vi "OCT with WavePond Clock periodic save.vi"() -> ()   [LabVIEW 2014]
doc: "I. Description:\nThis example demonstrates how to acquire a continuous amount of data (Waveform) using the DAQ device's internal clock.\n\nII. Instructions for Running:\n1. Create an analog input voltage channel.\n2. Set the rate for the sample clock. Additionally, define the sample mode to be continuous.\n3. Call the Start VI to start the acquisition.\n4. Read the waveform data in a loop until the user hits the stop button or an error occurs.\nNote: This example reads data from one or more channels and returns an array of data. Use the Index Array function to access an individual channel of data.\n5. Call the Clear Task VI to clear the Task.\n6. Use the popup dialog box to display an error if any.\n\nIV. I/O Connections Overview:\nMake sure your signal input terminal matches the Physical Channel I/O Control. For further connection information, refer to your hardware reference manual."
uses:
  ATS-VI/ATS_ctl/Device_Ctrl.ctl
  ATS-VI/ATS_ctl/ATS_Async_Ctrl.ctl
  ATS-VI/ATS_ctl/ATS_Async_Mode.ctl
  ATS-VI/ATS_ctl/ATS_DMA_Channel.ctl
  ATS-VI/ATS_ctl/ATS_ReadSamples.ctl
  ATS-VI/ATS_ctl/ATS_Check_Ctrl.ctl
  ATS-VI/ATS_ctl/ClockSource.ctl
  Galvo VIs/galvo_states.ctl
  Signal Processing/processing_states.ctl
  En Face/En Face States.ctl
  Saving Data/Saving Data States.ctl
  Type Defs/OCT Hardware States.ctl
  ATS-VI/ATS_ctl/Range.ctl
  ATS-VI/ATS_ctl/Impedance.ctl
  Type Defs/OCT Imaging Parameters Cluster.ctl
  Signal Processing/Display Raw Data states.ctl
  ATS-VI/ATS_ctl/ATS_Spec_Selector.ctl
  Classes/Galvo/Scanning Cluster.ctl
  Classes/Galvo/Galvo.lvclass
  Type Defs/OCT DAQ Channel Data Type.ctl
  Type Defs/Display States.ctl
  ATS-VI/ATS_ctl/Coupling.ctl
  ATS-VI/ATS_ctl/Bandwidth.ctl
  ATS-VI/ATS_ctl/InputCtrl.ctl
  ATS-VI/ATS_ctl/TriggerEngine.ctl
  ATS-VI/ATS_ctl/ExtTrigRange.ctl
  ATS-VI/ATS_ctl/ExtTrigger.ctl
  ATS-VI/ATS_ctl/TriggerOperation.ctl
  ATS-VI/ATS_ctl/Trigger.ctl
  ATS-VI/ATS_ctl/ClockRate.ctl
  ATS-VI/ATS_ctl/ClockEdge.ctl
  ATS-VI/ATS_ctl/Clock.ctl
  ATS-VI/ATS_ctl/Record.ctl
  ATS-VI/ATS_ctl/ATS_Global.ctl
  ATS-VI/ATS_ctl/ATS_Async_Status.ctl
  En Face/En Face Depth Parameters.ctl
  ATS-VI/ATS_ctl/ATS_Async_Setting.ctl
panel:
  in  "update en face image?":bool
  in  "total measurement time":dbl
  in  "save every ? second":dbl
  out "First Time?":bool
  out "Save Data":bool
  in  "Async_Setting":T1
  out "Processing Finished":bool
  in  "OCT Hardware States":T2=enum."Save Sweep"
  out "Save State":T3=enum."Initialize"
  out "Clock Length":u32=6304
  out "Reset DAQ":bool
  in  "Tab Control":T4(tab)
  in  "B-Scans Per Buffer":i32=4
  out "Async_Status":T5
  out "Current State":T2=enum."Set Resampling Array"
  in  "Channels":tag="Dev1/ao0:1"
  in  "Trigger Source":tag="/Dev1/PFI7"
  in  "Imaging Parameters":T6={"Points Per A-Scan"=0, "A-Scans per B-Scan"=0, "Voltage Range"=1.0, "Card Resolution (bits)"=12}
  in  "Setup_In":T7={"Record"={"Count"=1, "Presize"=0, "Length"=1408}, "Clock"={"ClckSource"=enum."External", "ClckRate"=17, "ClckEdge"=0, "Decimation"=0}, "Input A"={"Coupling"=enum."DC", "Range"=3, "Impedance"=enum."50 ohms", "Bandwidth"=enum."Full Bandwidth"}, "Input B"={"Coupling"=enum."DC", "Range"=3, "Impedance"=enum."50 ohms", "Bandwidth"=enum."Full Bandwidth"}, "Trigger"={"TrigOperation"=enum."Only X", "Timeout (s)"=1.0, "Trig. Delay"=0, "Engine X"={"Source"=enum."External", "Slope"=enum."Positive", "Level"=150}, "Engine Y"={"Source"=enum."Disable", "Slope"=enum."Positive", "Level"=128}, "ExtTrigControl"={"Coupling"=enum."DC", "Range"=enum."TTL"}}} {"Clock"."ClckEdge" items=["Rising", "Falling"]; "Clock"."ClckRate" items=["1 kS/s", "2 kS/s", "5 kS/s", "10 kS/s", "20 kS/s", "50 kS/s", "100 kS/s", "200 kS/s", "500 kS/s", "1 MS/s", "2 MS/s", "5 MS/s", "10 MS/s", "20 MS/s", "50 MS/s", "100 MS/s", "125 MS/s", "160 MS/s", "180 MS/s"]; "Input B"."Range" items=["200mV", "400mV", "800mV", "2 V", "4 V", "8 V", "16 V"]; "Trigger"."Timeout (s)" format="%.2f"; "Input A"."Range" items=["200mV", "400mV", "800mV", "2 V", "4 V", "8 V", "16 V"]}
  in  "OK Button":bool
  in  "Data Format":T23
  out "Channel A or B Phase (or Channel B Raw)":sgl[][](graph)
  out "Channel A or B Intensity (or Channel A Raw)":sgl[][](graph)
  in  "Display":T24
  out "En Face":dbl[][](graph)
  in  "En Face Parameters":T25={"En Face Start\nDepth"=50, "En Face End\nDepth"=200}
  in  "Save Sweep":bool
  in  "Scanning":T26={"Fast Axis Offset"=300.0, "Slow Axis Offset"=1.0, "Slow Axis Amp"=8.0, "Fast Axis Amp"=8.0, "B-scans (rings)"=1, "A(cluster)/B"=0, "Scan Pattern"=enum."Raster"} {"A(cluster)/B" max=1000 step=1; "B-scans (rings)" max=1000 step=1; "Fast Axis Amp" max=20 format="%#.2f"; "Slow Axis Amp" max=20 format="%#.2f"; "Slow Axis Offset" max=10 format="%#.2f"; "Fast Axis Offset" max=10 format="%#.2f"}
  in  "Stop Button":bool
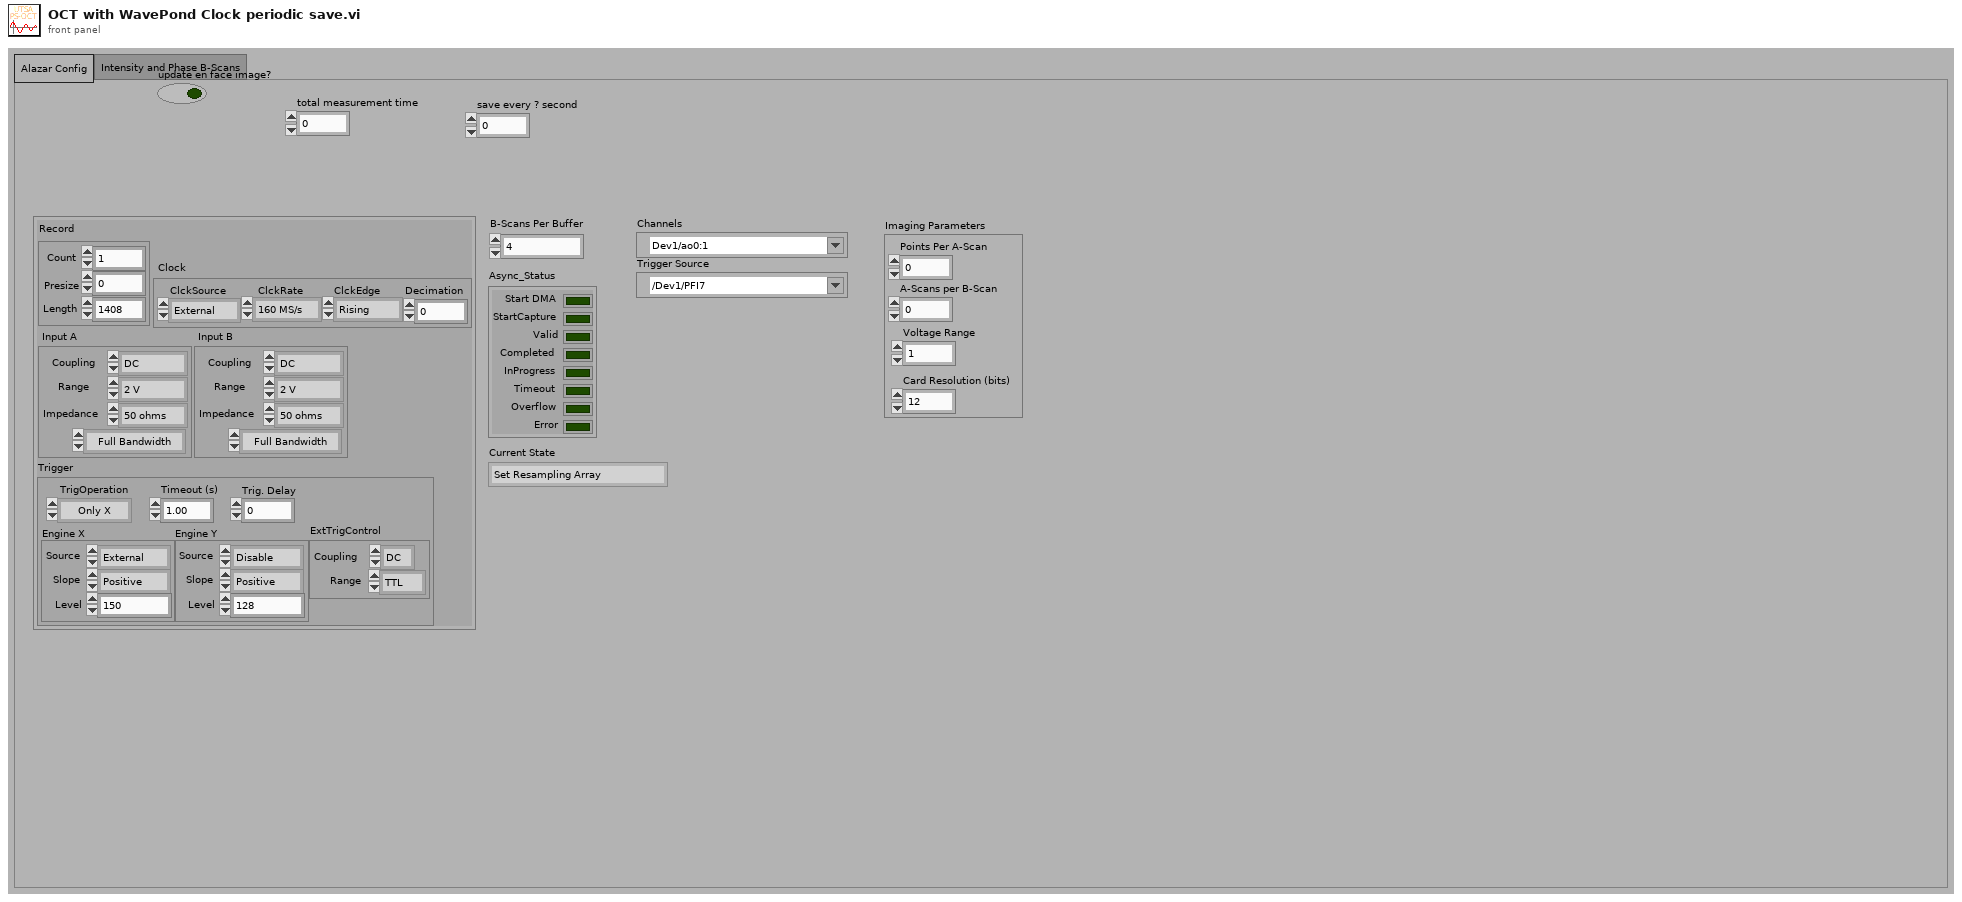
[diagram p1: front panel]
types:
  T1 = typedef "ATS_Async_Setting.ctl" = cluster{"UseHeader":u32, "Rec/Buffer":u32, "Total_Rec":u32, "DataBuffer":bool, "GetProcessedData":bool}
  T2 = typedef "OCT Hardware States.ctl" = enum16{"Acquire Data", "Initialize Laser", "Initialize Galvos", "Startup", "Reset DAQ", "Background Subtraction", "Acquire Background", "Update DAQ Parameters", "Stop", "Set Clock", "Initialize DAQ", "Set Resampling Array", "Save Sweep", "Configure Laser", "128 x 128", "512 x 512", "Review Data"}
  T3 = typedef "Saving Data States.ctl" = enum16{"Get Queue Size", "Get Queue", "Get Timeout", "Flush Queue", "Close Files", "Create Files", "Do Nothing", "Initialize", "Enqueue Data", "Save Data", "Shutdown"}
  T4 = enum32{"Alazar Config", "Intensity and Phase B-Scans"}
  T5 = typedef "ATS_Async_Status.ctl" = cluster{"Start DMA":bool, "StartCapture":bool, "Valid":bool, "Completed":bool, "InProgress":bool, "Timeout":bool, "Overflow":bool, "Error":bool}
  T6 = typedef "OCT Imaging Parameters Cluster.ctl" = cluster{"Points Per A-Scan":i32, "A-Scans per B-Scan":i32, "Voltage Range":sgl, "Card Resolution (bits)":u16}
  T7 = typedef "ATS_Global.ctl" = cluster{"Record":T8, "Clock":T9, "Input A":T13, "Input B":T13, "Trigger":T18}
  T8 = typedef "Record.ctl" = cluster{"Count":u32, "Presize":u32, "Length":u32}
  T9 = typedef "Clock.ctl" = cluster{"ClckSource":T10, "ClckRate":T11, "ClckEdge":T12, "Decimation":u32}
  T10 = typedef "ClockSource.ctl" = enum16{"Internal", "External", "Medium Ext.", "Slow Ext.", "Ext. AC", "Ext. DC", "Ext. (PLL)"}
  T11 = typedef "ClockRate.ctl" = u32
  T12 = typedef "ClockEdge.ctl" = u16
  T13 = typedef "InputCtrl.ctl" = cluster{"Coupling":T14, "Range":T15, "Impedance":T16, "Bandwidth":T17}
  T14 = typedef "Coupling.ctl" = enum16{"AC", "DC"}
  T15 = typedef "Range.ctl" = u32
  T16 = typedef "Impedance.ctl" = enum16{"1M ohms", "50 ohms"}
  T17 = typedef "Bandwidth.ctl" = enum16{"Full Bandwidth", "Reduce Bandwidth"}
  T18 = typedef "Trigger.ctl" = cluster{"TrigOperation":T19, "Timeout (s)":dbl, "Trig. Delay":u32, "Engine X":T20, "Engine Y":T20, "ExtTrigControl":T21}
  T19 = typedef "TriggerOperation.ctl" = enum16{"Only X", "Only Y", "X or Y", "X and Y", "X xor Y", "X and not Y", "not X and Y"}
  T20 = typedef "TriggerEngine.ctl" = cluster{"Source":enum32{"Chan_A", "Chan_B", "External", "Disable"}, "Slope":enum32{"Positive", "Negative"}, "Level":u32}
  T21 = typedef "ExtTrigger.ctl" = cluster{"Coupling":T14, "Range":T22}
  T22 = typedef "ExtTrigRange.ctl" = enum16{"1 V", "5 V", "TTL"}
  T23 = typedef "OCT DAQ Channel Data Type.ctl" = enum16{"Channel 1", "Channel 2", "Channel 1 and 2"}
  T24 = typedef "Display States.ctl" = enum16{"Channel A", "Channel B"}
  T25 = typedef "En Face Depth Parameters.ctl" = cluster{"En Face Start\nDepth":i32, "En Face End\nDepth":i32}
  T26 = typedef "Galvo.lvclass/Scanning Cluster.ctl" = cluster{"Fast Axis Offset":sgl, "Slow Axis Offset":sgl, "Slow Axis Amp":sgl, "Fast Axis Amp":sgl, "B-scans (rings)":u32, "A(cluster)/B":u32, "Scan Pattern":enum16{"Raster"}}
  T27 = typedef "ATS_Check_Ctrl.ctl" = enum16{"None", "NO_ATS9462", "ATS9462_Traditional", "Verify Board", "OnBoard Memory", "Board & Memory", "Master/Slave", "NO Master/Slave"}
  T28 = typedef "Device_Ctrl.ctl" = enum16{"Status", "About", "Arm", "ForceTrig", "Abort", "Initialize", "Init (NoPreset)", "Info", "Close", "Calibrate", "SetManually", "LED_ON", "LED_OFF"}
  T29 = typedef "ATS_Spec_Selector.ctl" = enum16{"None", "ClckSource", "ClckEdge", "ClckRate", "InputRange", "InputCoupling", "Impedance", "Bandwidth", "AsyncDMA", "Memory", "ExtTrigCoupling", "ExtTrigRange", "AUX_IO_Trig", "AUX_IO_Slope", "Trigger_Source"}
  T30 = typedef "galvo_states.ctl" = enum16{"Reset", "Reset Galvos?", "Center Galvos", "Register Callback", "Get Scan Parameters", "Show", "Initialize", "Run Raster", "Load Raster", "Run Circle", "Shutdown"}
  T31 = typedef "processing_states.ctl" = enum16{"Initialize", "Set Background", "Update Imaging Parameters", "Get Queue", "Process Data", "Get Size", "Flush Data", "Set Reample Array", "Get Last Processed BScan", "Shutdown"}
  T32 = typedef "Display Raw Data states.ctl" = enum16{"Add Raw", "Add Processed", "Show"}
  T33 = typedef "En Face States.ctl" = enum16{"Save BMP", "Show", "Clear En Face", "Update EnFace"}
  T34 = typedef "Processed OCT Data.ctl" = cluster{"Intensity A":sgl[][][], "Phase A":sgl[][][], "Intensity B":sgl[][][], "Phase B":sgl[][][]}
  T35 = enum8{"Enabled", "Disabled", "Disabled and Grayed Out"}
  T36 = typedef "ATS_Async_Ctrl.ctl" = enum16{"SetupDMA", "StartCapture", "Get", "Get_Stream", "Abort", "Stop"}
  T37 = typedef "ATS_ReadSamples.ctl" = cluster{"Offset":i32, "Length":u32}
  T38 = typedef "ATS_DMA_Channel.ctl" = enum16{"Channel_A", "Channel_B", "A & B"}
  T39 = typedef "ATS_Async_Mode.ctl" = enum16{"Continuous", "Triggered", "No-Pre-Trigger", "Traditional"}
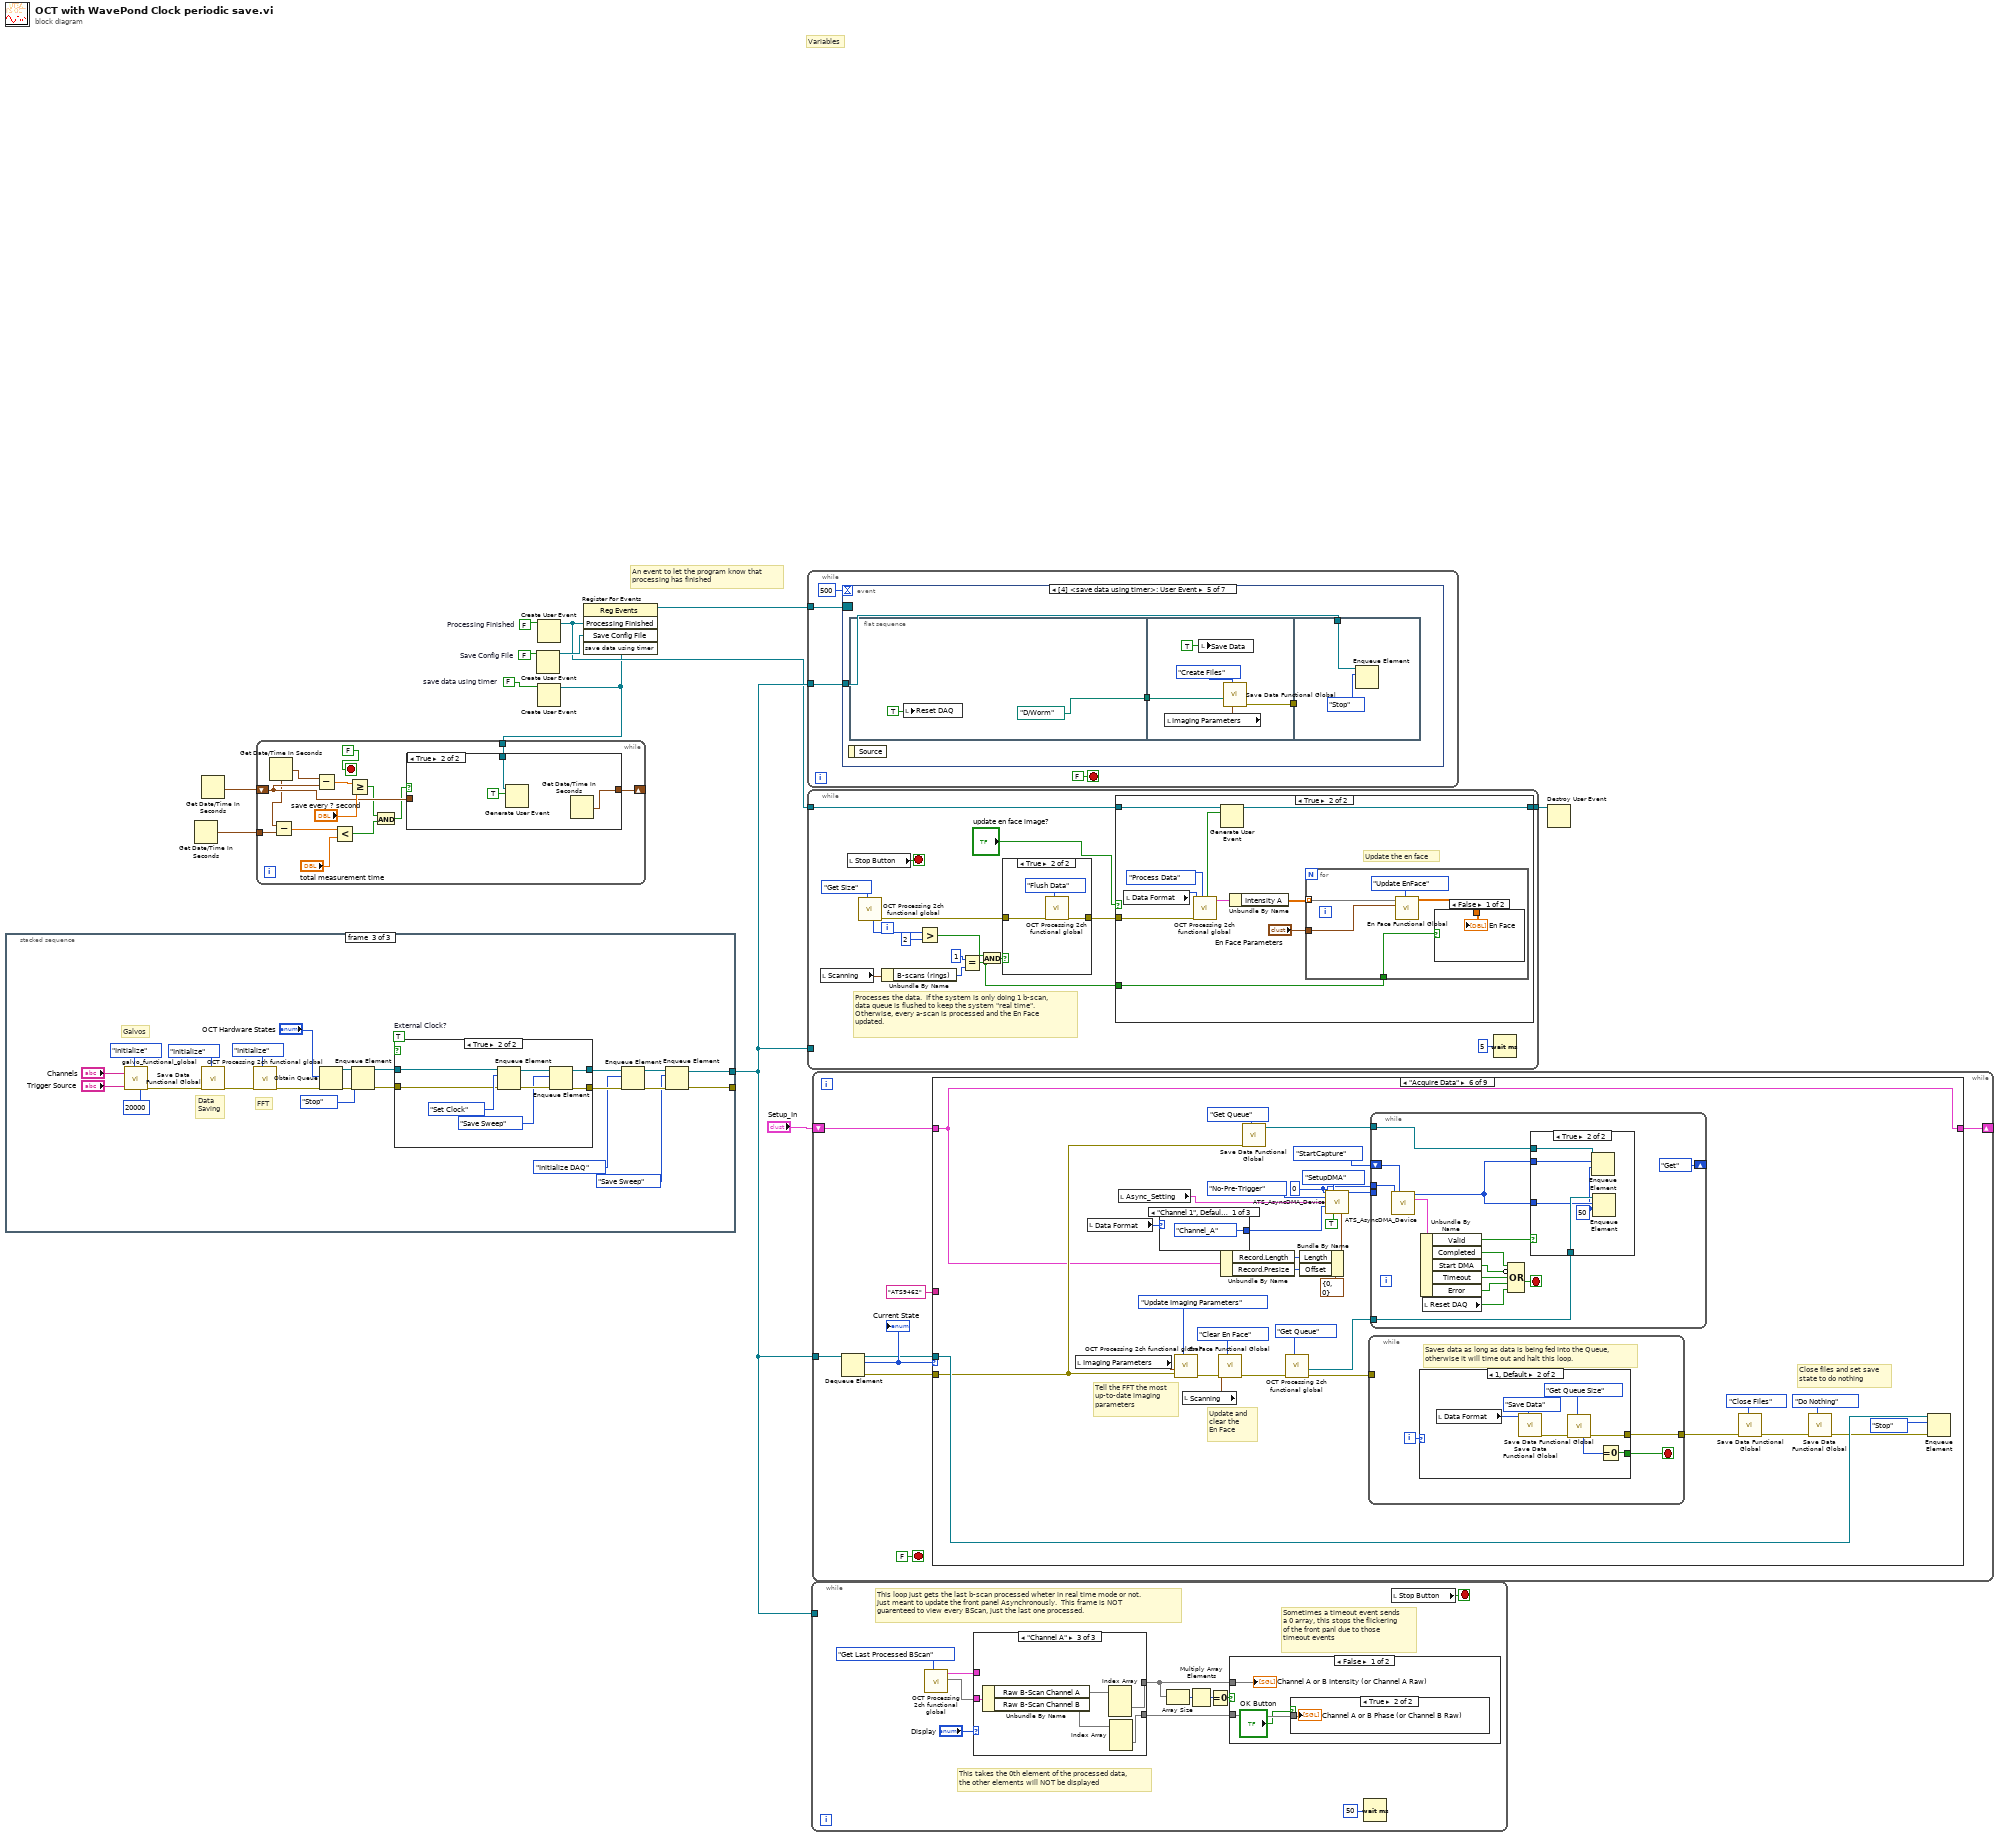
[diagram p0: block diagram]
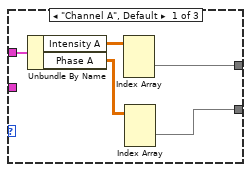
[diagram p8: hidden frame]
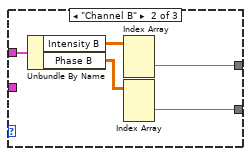
[diagram p9: hidden frame]
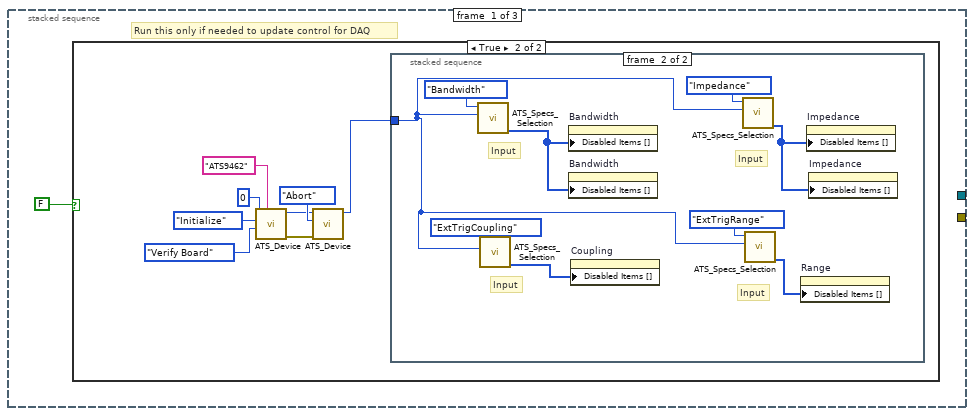
[diagram p10: hidden frame]
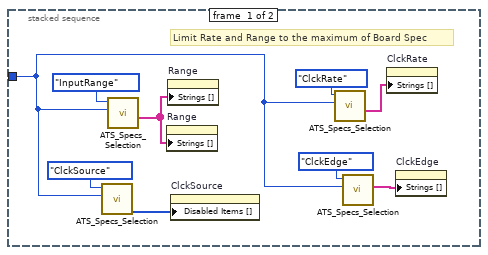
[diagram p12: hidden frame]
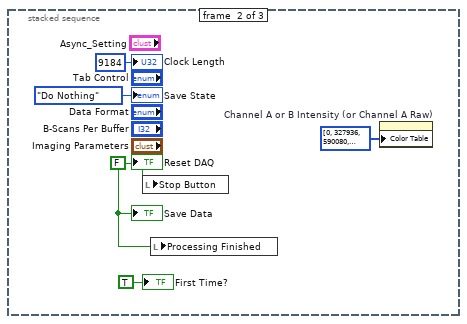
[diagram p13: hidden frame]
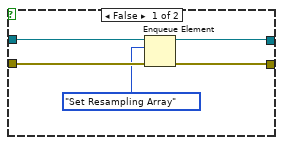
[diagram p14: hidden frame]
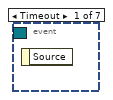
[diagram p15: hidden frame]
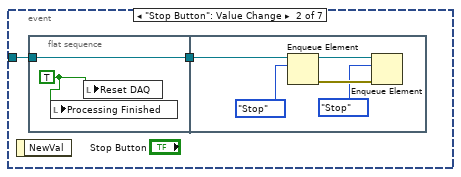
[diagram p16: hidden frame]
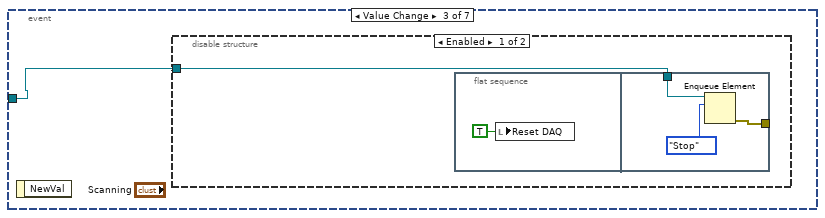
[diagram p17: hidden frame]
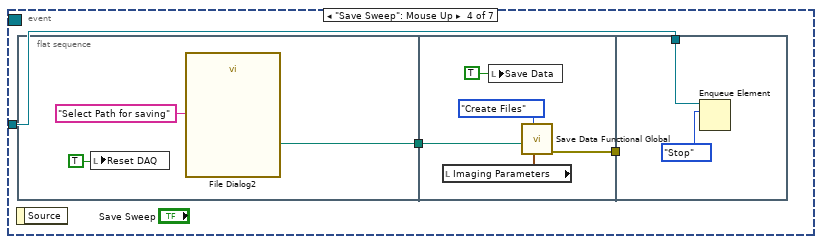
[diagram p19: hidden frame]
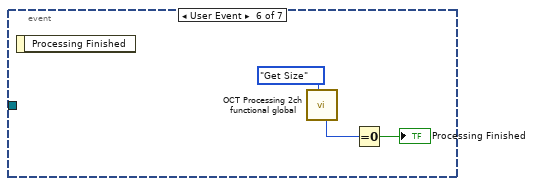
[diagram p20: hidden frame]
diagram:
  w3 = FALSE  # save data using timer
  w4 = FALSE  # Save Config File
  w12 = FALSE  # Processing Finished
  # "An event to let the program know that\nprocessing has finished"
  # "Variables"
  n1 = stacked-sequence {
    tunnel: [_ _ w58] -> _
    tunnel: [_ _ w64] -> w9
    frame #0 {
      # "Run this only if needed to update control for DAQ"
      n2 = case shown="True" FALSE {
        frame False {
        }
        frame True {
          n3 = call "ATS_Device.vi"("BoardToVerify"="ATS9462", "ATS_Check"=ATS_Check_Ctrl."Verify Board", "DevCtrl"=Device_Ctrl."Initialize", "DeviceIn"=0 ("Device")) -> ("error out"=w17:errorcluster, "DeviceOut"=w19:i32)  [unwired: 1 in, 5 out]
          n4 = call "ATS_Device.vi"("error in (no error)"=w17, "DevCtrl"=Device_Ctrl."Abort", "DeviceIn"=w19) -> ("DeviceOut"=w15:i32)  [unwired: 2 in, 6 out]
          n5 = stacked-sequence {
            tunnel: w15 -> [w24 w31]
            frame #0 {
              # "Limit Rate and Range to the maximum of Board Spec"
              n6 = call "ATS_Specs_Selection.vi"("Device"=w24, "ATS_Spec_Selector"=ATS_Spec_Selector."ClckSource") -> ("Disabled_Item"=w23:i32[])  [unwired: 3 in, 6 out]
              n7 = call "ATS_Specs_Selection.vi"("Device"=w24, "ATS_Spec_Selector"=ATS_Spec_Selector."InputRange") -> ("Possible_Item"=w30:string[])  [unwired: 3 in, 6 out]
              n8 = property on="Range" class="Ring (strict)"("Strings []"=w30) -> ()  [unwired: 2 in, 2 out]
              n9 = property on="Range" class="Ring (strict)"("Strings []"=w30) -> ()  [unwired: 2 in, 2 out]
              n10 = property on="ClckSource" class="Enum (strict)"("Disabled Items []"=w23) -> ()  [unwired: 2 in, 2 out]
              n11 = call "ATS_Specs_Selection.vi"("Device"=w24, "ATS_Spec_Selector"=ATS_Spec_Selector."ClckRate") -> ("Possible_Item"=w28:string[])  [unwired: 3 in, 6 out]
              n12 = call "ATS_Specs_Selection.vi"("Device"=w24, "ATS_Spec_Selector"=ATS_Spec_Selector."ClckEdge") -> ("All_Item"=w22:string[])  [unwired: 3 in, 6 out]
              n13 = property on="ClckRate" class="Ring (strict)"("Strings []"=w28) -> ()  [unwired: 2 in, 2 out]
              n14 = property on="ClckEdge" class="Ring (strict)"("Strings []"=w22) -> ()  [unwired: 2 in, 2 out]
            }
            frame #1 {
              # "Input"
              # "Input"
              # "Input"
              # "Input"
              n15 = call "ATS_Specs_Selection.vi"("Device"=w31, "ATS_Spec_Selector"=ATS_Spec_Selector."Bandwidth") -> ("Disabled_Item"=w37:i32[])  [unwired: 3 in, 6 out]
              n16 = call "ATS_Specs_Selection.vi"("Device"=w31, "ATS_Spec_Selector"=ATS_Spec_Selector."ExtTrigCoupling") -> ("Disabled_Item"=w33:i32[])  [unwired: 3 in, 6 out]
              n17 = property on="Bandwidth" class="Enum (strict)"("Disabled Items []"=w37) -> ()  [unwired: 2 in, 2 out]
              n18 = property on="Bandwidth" class="Enum (strict)"("Disabled Items []"=w37) -> ()  [unwired: 2 in, 2 out]
              n19 = property on="Coupling" class="Enum (strict)"("Disabled Items []"=w33) -> ()  [unwired: 2 in, 2 out]
              n20 = call "ATS_Specs_Selection.vi"("Device"=w31, "ATS_Spec_Selector"=ATS_Spec_Selector."Impedance") -> ("Disabled_Item"=w36:i32[])  [unwired: 3 in, 6 out]
              n21 = call "ATS_Specs_Selection.vi"("Device"=w31, "ATS_Spec_Selector"=ATS_Spec_Selector."ExtTrigRange") -> ("Disabled_Item"=w32:i32[])  [unwired: 3 in, 6 out]
              n22 = property on="Range" class="Enum (strict)"("Disabled Items []"=w32) -> ()  [unwired: 2 in, 2 out]
              n23 = property on="Impedance" class="Enum (strict)"("Disabled Items []"=w36) -> ()  [unwired: 2 in, 2 out]
              n24 = property on="Impedance" class="Enum (strict)"("Disabled Items []"=w36) -> ()  [unwired: 2 in, 2 out]
            }
          }
        }
      }
    }
    frame #1 {
      w41 = FALSE ("Sweep Ready for saving")
      n25 = local write "Stop Button"(w41) -> ()
      n26 = local write "Processing Finished"(w41) -> ()
      n27 = property on="Channel A or B Intensity (or Channel A Raw)" class="IntGraph (strict)"("Color Table"=u32[] [0, 327936, 590080, 852224, 983296, 1114624, 1180160, 1311232, 1442304, 1573632, 1704704, 1770240, 1901312, 1966848, 2098176, 2163712, 2294784, 2491392, 2557184, 2688256, 2753792, 2884864, 2950656, 3081728, 3147264, 3344129, 3475457, 3540993, 3672321, 3738113, 3869185, 3934977, 4066305, 4197633, 4328961, 4394497, 4460289, 4591617, 4657409, 4788481, 4854273, 4985601, 5116929, 5248257, 5314049, 5379841, 5511169, 5576961, 5708033, 5773825, 5905153, 6036482, 6167810, 6233346, 6299138, 6430466, 6496258, 6562050, 6693634, 6759426, 6890754, 7022082, 7087874, 7153666, 7284994, 7350786, 7482114, 7547906, 7613698, 7745026, 7876354, 8007682, 8073474, 8139522, 8205314, 8336642, 8467970, 8533763, 8599555, 8665347, 8731139, 8862467, 8993795, 9059587, 9125380, 9191428, 9257220, 9388548, 9454340, 9520132, 9585924, 9717253, 9848837, 9914629, 9980165, 10045957, 10177541, 10243334, 10309126, 10375174, 10440966, 10572294, 10703623, 10769416, 10835208, 10901256, 10967049, 11033097, 11033609, 11099401, 11165450, 11231242, 11231754, 11297547, 11363339, 11429131, 11495180, 11495692, 11561740, 11693069, 11758861, 11759373, 11825165, 11891214, 11957006, 12022799, 12023311, 12089103, 12220944, 12286736, 12286736, 12352529, 12418577, 12484370, 12550162, 12615954, 12681747, 12747796, 12813588, 12813845, 12879894, 12945686, 13077015, 13142808, 13143064, 13208856, 13274905, 13340697, 13340953, 13472282, 13538075, 13604379, 13670172, 13735964, 13801757, 13867550, 13933343, 13999392, 13999648, 14065441, 14131234, 14197027, 14197541, 14263334, 14329383, 14395176, 14460969, 14592553, 14658346, 14724139, 14789932, 14790189, 14856238, 14922287, 14988080, 15053873, 15054130, 15119923, 15185972, 15251765, 15317559, 15383353, 15449146, 15449660, 15515454, 15515968, 15516226, 15582021, 15582278, 15582536, 15648587, 15648844, 15714639, 15714897, 15715155, 15780949, 15781463, 15847256, 15847770, 15848028, 15913823, 15914081, 15979875, 15980133, 15980391, 16046441, 16046444, 16046703, 16046705, 16112500, 16113015, 16113274, 16113277, 16179072, 16179330, 16179588, 16245384, 16245387, 16245389, 16245648, 16311443, 16376982, 16377241, 16377499, 16443294, 16443553, 16443555, 16443815, 16509866, 16510124, 16510127, 16575923, 16575924, 16576182, 16576441, 16576443, 16576702, 16576705, 16576963, 16577222, 16577224, 16577482, 16577485, 16577743, 16577745, 16578004, 16578262, 16578264, 16578523, 16578782, 16579040, 16579299, 16579301, 16579303, 16579562, 16579821]) -> ()  [unwired: 2 in, 2 out]
      "Clock Length" <- u32 9184 ("Clock Length")
      "Save State" <- Saving_Data_States."Do Nothing" ("Save State")
      "Reset DAQ" <- w41
      "Save Data" <- w41
      "First Time?" <- TRUE ("First Time?")
    }
    frame #2 {
      w46 = TRUE  # External Clock?
      # "FFT"
      # "Data \nSaving"
      # "Galvos"
      n28 = call "galvo_functional_global.vi"(4:20000 ("Sweep Speed"), "State"=galvo_states."Initialize", "Trigger Source"="Trigger Source", "Analog Output"="Channels") -> ("error out"=w55:errorcluster)  [unwired: 6 in, 1 out]
      n29 = call "Save Data Functional Global.vi"("States"=Saving_Data_States."Initialize", "error in (no error)"=w55) -> ("error out"=w60:errorcluster)  [unwired: 6 in, 3 out]
      n30 = call "OCT Processing 2ch functional global.vi"("State"=processing_states."Initialize", "error in (no error)"=w60) -> ("error out"=w61:errorcluster)  [unwired: 5 in, 4 out]
      n31 = Obtain Queue(element data type="OCT Hardware States", error in (no error)=w61) -> (queue out=w49:refnum<queue>, error out=w48:errorcluster)  [unwired: 3 in, 1 out]
      n32 = Enqueue Element(queue=w49, element=OCT_Hardware_States."Stop", error in (no error)=w48) -> (queue out=w51:refnum<queue>, error out=w50:errorcluster)  [unwired: 1 in, 1 out]
      n33 = case shown="True" w46 {
        tunnel: [w70 w79] -> w68
        tunnel: [w71 w78] -> w67
        tunnel: w51 -> [w73 w75]
        tunnel: w50 -> [w72 w74]
        frame False {
          n34 = Enqueue Element(queue=w73, element=OCT_Hardware_States."Set Resampling Array", error in (no error)=w72) -> (queue out=w70:refnum<queue>, error out=w71:errorcluster)  [unwired: 1 in, 1 out]
        }
        frame True {
          n35 = Enqueue Element(queue=w75, element=OCT_Hardware_States."Set Clock", error in (no error)=w74) -> (queue out=w81:refnum<queue>, error out=w80:errorcluster)  [unwired: 1 in, 1 out]
          n36 = Enqueue Element(queue=w81, element=OCT_Hardware_States."Save Sweep", error in (no error)=w80) -> (queue out=w79:refnum<queue>, error out=w78:errorcluster)  [unwired: 1 in, 1 out]
        }
      }
      n37 = Enqueue Element(queue=w68, element=OCT_Hardware_States."Initialize DAQ", error in (no error)=w67) -> (queue out=w66:refnum<queue>, error out=w65:errorcluster)  [unwired: 1 in, 1 out]
      n38 = Enqueue Element(queue=w66, element=OCT_Hardware_States."Save Sweep", error in (no error)=w65) -> (queue out=w64:refnum<queue>, error out=w58:errorcluster)  [unwired: 1 in, 1 out]
    }
  }
  n39 = Get Date/Time In Seconds() -> (seconds since 1Jan1904=w1:timestamp)
  n40 = Get Date/Time In Seconds() -> (seconds since 1Jan1904=w5:timestamp)
  n41 = Create User Event(user event datatype=w4) -> (user event=w8:refnum<user-event>)  [unwired: 1 in, 1 out]
  n42 = Create User Event(user event datatype=w12) -> (user event=w7:refnum<user-event>)  [unwired: 1 in, 1 out]
  n43 = Create User Event(user event datatype=w3) -> (user event=w2:refnum<user-event>)  [unwired: 1 in, 1 out]
  n44 = while {
    shift-right: [w91] -> _
    shift-left: w5 -> [w90]
    tunnel: w2 -> [w89]
    tunnel: w1 -> [w87]
    stop <- FALSE stop-if-true
    n45 = Get Date/Time In Seconds() -> (seconds since 1Jan1904=w86:timestamp)
    n46 = Subtract(x=w86, y=w87) -> (x-y=w85:dbl)
    n47 = Subtract(x=w86, y=w90) -> (x-y=w93:dbl)
    n48 = Less?(x=w85, y="total measurement time") -> (x < y?=w84:bool)
    n49 = Greater Or Equal?(x=w93, y="save every ? second") -> (x >= y?=w83:bool)
    n50 = And(x=w83, y=w84) -> (x .and. y?=w82:bool)
    n51 = case shown="True" w82 {
      tunnel: [w95 w98] -> w91
      tunnel: w90 -> [w95 _]
      tunnel: w89 -> [_ w97]
      frame False {
      }
      frame True {
        n52 = Generate User Event(user event=w97, event data cluster=TRUE ("event data")) -> ()  [unwired: 2 in, 2 out]
        n53 = Get Date/Time In Seconds() -> (seconds since 1Jan1904=w98:timestamp)
      }
    }
  }
  n54 = register-events(w7, w8, w2) -> (reference out=w11:refnum<event-registration>)  [unwired: 2 in, 1 out]
  n55 = while {
    tunnel: w9 -> [w100]
    tunnel: w11 -> [w101]
    stop <- FALSE stop-if-true
    n56 = event shown="[4] <save data using timer>: User Event" {
      selector: w101 -> [_ _ _ _ _ _ _]
      dyn-events: _ -> [_ _ _ _ _ _ _]
      timeout: 500 -> [_ _ _ _ _ _ _]
      tunnel: w100 -> [_ w103 w112 w120 w133 _ _]
      event Timeout {
        n57 = event-data() -> ()  [unwired: 1 in, 1 out]
      }
      event "Stop Button": Value Change {
        n58 = event-data() -> ()  [unwired: 1 in, 1 out]
        n59 = flat-sequence {
          tunnel: w103 -> [w106]
          tunnel: [w106] -> w104
          tunnel: w104 -> [w111]
          frame #0 {
            w105 = TRUE ("Reset DAQ")
            n60 = local write "Processing Finished"(w105) -> ()
            n61 = local write "Reset DAQ"(w105) -> ()
          }
          frame #1 {
            n62 = Enqueue Element(queue=w111, element=OCT_Hardware_States."Stop") -> (queue out=w108:refnum<queue>, error out=w109:errorcluster)  [unwired: 2 in, 1 out]
            n63 = Enqueue Element(queue=w108, element=OCT_Hardware_States."Stop", error in (no error)=w109) -> ()  [unwired: 1 in, 3 out]
          }
        }
      }
      event Value Change {
        n64 = event-data() -> ()  [unwired: 1 in, 1 out]
        n65 = disable-structure shown="Enabled" {
          disable-tunnel: w112 -> [w113 _]
          frame Enabled {
            n66 = flat-sequence {
              tunnel: w113 -> [w116]
              tunnel: [w115] -> _
              frame #0 {
                n67 = local write "Reset DAQ"(TRUE ("Reset DAQ")) -> ()
              }
              frame #1 {
                n68 = Enqueue Element(queue=w116, element=OCT_Hardware_States."Stop") -> (error out=w115:errorcluster)  [unwired: 2 in, 2 out]
              }
            }
          }
          frame Disabled {
          }
        }
      }
      event "Save Sweep": Mouse Up {
        n69 = event-data() -> ()  [unwired: 1 in, 1 out]
        n70 = flat-sequence {
          tunnel: [w121] -> w119
          tunnel: w119 -> [w128]
          tunnel: [w126] -> w118
          tunnel: w120 -> [w130]
          tunnel: w118 -> [_]
          frame #0 {
            n71 = local write "Reset DAQ"(TRUE ("Reset DAQ")) -> ()
            n72 = call "File Dialog2"("prompt"="Select Path for saving") -> ("selected path"=w121:path)  [unwired: 11 in, 3 out]
          }
          frame #1 {
            n73 = local read "Imaging Parameters"() -> (w125:T6)
            n74 = local write "Save Data"(TRUE ("Save Data")) -> ()
            n75 = call "Save Data Functional Global.vi"("Input Parameters"=w125, "States"=Saving_Data_States."Create Files", "Folder"=w128) -> ("error out"=w126:errorcluster)  [unwired: 5 in, 3 out]
          }
          frame #2 {
            n76 = Enqueue Element(queue=w130, element=OCT_Hardware_States."Stop") -> ()  [unwired: 2 in, 3 out]
          }
        }
      }
      event User Event {
        n77 = event-data() -> ()  [unwired: 1 in, 1 out]
        n78 = flat-sequence {
          tunnel: [path "D:/Worm" ("selected path")] -> w132
          tunnel: w132 -> [w140]
          tunnel: [w138] -> w131
          tunnel: w133 -> [w142]
          tunnel: w131 -> [_]
          frame #0 {
            n79 = local write "Reset DAQ"(TRUE ("Reset DAQ")) -> ()
          }
          frame #1 {
            n80 = local read "Imaging Parameters"() -> (w137:T6)
            n81 = local write "Save Data"(TRUE ("Save Data")) -> ()
            n82 = call "Save Data Functional Global.vi"("Input Parameters"=w137, "States"=Saving_Data_States."Create Files", "Folder"=w140) -> ("error out"=w138:errorcluster)  [unwired: 5 in, 3 out]
          }
          frame #2 {
            n83 = Enqueue Element(queue=w142, element=OCT_Hardware_States."Stop") -> ()  [unwired: 2 in, 3 out]
          }
        }
      }
      event User Event {
        n84 = event-data() -> ()  [unwired: 1 in, 1 out]
        n85 = call "OCT Processing 2ch functional global.vi"("State"=processing_states."Get Size") -> ("# elements in queue"=w144:i32)  [unwired: 6 in, 4 out]
        n86 = Equal To 0?(x=w144) -> (x = 0?=→"Processing Finished":bool)
      }
      event Menu Selection (User) {
        n87 = event-data() -> ("ItemTag"=w146:string)  [unwired: 1 in, 2 out]
        n88 = case shown="\"Raw Data\", Default" w146 {
          frame "Raw Data", Default {
            n89 = call "Display Raw Data.vi"("Enum"=Display_Raw_Data_states."Show") -> ()  [unwired: 11 in]
          }
        }
      }
    }
  }
  n90 = while {
    tunnel: w7 -> [w154]
    tunnel: [w153] -> w10
    tunnel: w9 -> [_]
    stop <- w163 stop-if-true
    # "Processes the data.  If the system is only doing 1 b-scan, \ndata queue is flushed to keep the system \"real time\".\nOtherwise, every a-scan is processed and the En Face\nupdated."
    n91 = local read "Scanning"() -> (w156:T26)
    n92 = local read "Stop Button"() -> (w163:bool)
    n93 = call "OCT Processing 2ch functional global.vi"("State"=processing_states."Get Size") -> ("error out"=w152:errorcluster, "# elements in queue"=w160:i32)  [unwired: 6 in, 3 out]
    n94 = Unbundle By Name(w156) -> ("B-scans (rings)"=w155:u32)
    n95 = Greater?(x=w160, y=2) -> (0:w161:bool)
    n96 = Equal?(x=u32 1, y=w155) -> (x = y?=w149:bool)
    n97 = And(x=w161, y=w149) -> (x .and. y?=w150:bool)
    n98 = case shown="True" w150 {
      tunnel: w152 -> [w181 w184]
      tunnel: [w181 w183] -> w151
      frame False {
      }
      frame True {
        n99 = call "OCT Processing 2ch functional global.vi"("State"=processing_states."Flush Data", "error in (no error)"=w184) -> ("error out"=w183:errorcluster)  [unwired: 5 in, 4 out]
      }
    }
    n100 = case shown="True" "update en face image?" {
      tunnel: w154 -> [w164 w171]
      tunnel: [w164 w169] -> w153
      tunnel: w151 -> [_ w166]
      tunnel: w149 -> [_ w165]
      frame False {
      }
      frame True {
        # "Update the en face"
        n101 = local read "Data Format"() -> (w172:T23)
        n102 = call "OCT Processing 2ch functional global.vi"("State"=processing_states."Process Data", "error in (no error)"=w166, "Data Format"=w172) -> ("Processed OCT Data"=w173:T34, "Time Out"=w170:bool)  [unwired: 4 in, 3 out]
        n103 = Generate User Event(user event=w171, event data cluster=w170) -> (user event out=w169:refnum<user-event>)  [unwired: 2 in, 1 out]
        n104 = Unbundle By Name(w173) -> ("Intensity A"=w167:sgl[][][])
        n105 = for {
          tunnel: "En Face Parameters" -> [w178]
          tunnel: w167 -> [w177] mode=indexing
          tunnel: w165 -> [w175]
          n106 = call "En Face Functional Global.vi"(7:En_Face_States."Update EnFace" ("En Face States"), 10:w178, "Intensity Graph 2"=w177) -> ("Intensity Graph"=w176:dbl[][])  [unwired: 7 in, 1 out]
          n107 = case shown="False" w175 {
            tunnel: w176 -> [w180 _]
            frame False {
              "En Face" <- w180
            }
            frame True {
            }
          }
        }
      }
    }
    n108 = Wait (ms)(milliseconds to wait=u32 5) -> ()  [unwired: 1 out]
  }
  n109 = while {
    tunnel: w9 -> [_]
    stop <- w195 stop-if-true
    # "Sometimes a timeout event sends\na 0 array, this stops the flickering\nof the front panl due to those \ntimeout events"
    # "This takes the 0th element of the processed data,\nthe other elements will NOT be displayed"
    # "This loop just gets the last b-scan processed wheter in real time mode or not. \nJust meant to update the front panel Asynchronously.  This frame is NOT\nguarenteed to view every BScan, just the last one processed."
    n110 = call "OCT Processing 2ch functional global.vi"("State"=processing_states."Get Last Processed BScan") -> (2:w191, "Processed OCT Data"=w189:T34)  [unwired: 5 in, 4 out]
    n111 = case shown="\"Raw Data A and B\"" "Display" {
      tunnel: w189 -> [w204 w205 _]
      tunnel: w191 -> [_ _ w214]
      tunnel: [w200 w207 w212] -> w187
      tunnel: [w201 w206 w211] -> w190
      frame "Channel A", Default {
        n112 = Unbundle By Name(w204) -> ("Intensity A"=w202:sgl[][][], "Phase A"=w203:sgl[][][])
        n113 = Index Array(array=w202) -> (element=w200:sgl[][])  [unwired: 3 in]
        n114 = Index Array(array=w203) -> (element=w201:sgl[][])  [unwired: 3 in]
      }
      frame "Channel B" {
        n115 = Unbundle By Name(w205) -> ("Intensity B"=w208:sgl[][][], "Phase B"=w209:sgl[][][])
        n116 = Index Array(array=w208) -> (element=w207:sgl[][])  [unwired: 3 in]
        n117 = Index Array(array=w209) -> (element=w206:sgl[][])  [unwired: 3 in]
      }
      frame "Channel A" {
        n118 = Unbundle By Name(w214) -> ("Raw B-Scan Channel A"=w210, "Raw B-Scan Channel B"=w213)
        n119 = Index Array(array=w210) -> (element=w212)  [unwired: 3 in]
        n120 = Index Array(array=w213) -> (element=w211)  [unwired: 3 in]
      }
    }
    n121 = Array Size(array=w187) -> (size(s)=w188:i32[])
    n122 = Multiply Array Elements(1:w188) -> (0:w186:i32)
    n123 = Equal To 0?(x=w186) -> (x = 0?=w185:bool)
    n124 = case shown="False" w185 {
      tunnel: w190 -> [w198 _]
      tunnel: w187 -> [w197 _]
      frame False {
        n125 = case shown="True" "OK Button" {
          tunnel: w198 -> [_ w199]
          frame False {
          }
          frame True {
            "Channel A or B Phase (or Channel B Raw)" <- w199
          }
        }
        "Channel A or B Intensity (or Channel A Raw)" <- w197
      }
      frame True {
      }
    }
    n126 = Wait (ms)(milliseconds to wait=u32 50) -> ()  [unwired: 1 out]
    n127 = local read "Stop Button"() -> (w195:bool)
  }
  n128 = while {
    tunnel: w9 -> [w222]
    shift-right: [w216] -> _
    shift-left: "Setup_In" -> [w215]
    stop <- FALSE stop-if-true
    n129 = Dequeue Element(queue=w222) -> (queue out=w218:refnum<queue>, element=w220:T2, error out=w219:errorcluster)  [unwired: 2 in, 1 out]
    "Current State" <- w220
    n130 = case shown="\"Acquire Data\"" w220 {
      tunnel: w219 -> [w236 w251 _ _ w353 w406 _ w481 _]
      tunnel: w218 -> [w235 w253 _ _ w362 w423 _ w482 _]
      tunnel: "ATS9462" ("BoardToVerify") -> [_ _ _ w314 _ _ _ _ w489]
      tunnel: [w234 w248 w264 w308 w349 w404 w471 w473 w488] -> w216
      tunnel: w215 -> [w234 w248 w264 w307 w349 w404 w471 w473 w488]
      frame "Save Sweep" {
        n131 = call "galvo_functional_global.vi"("State"=galvo_states."Reset", "error in (no error)"=w236) -> ("error out"=w224:errorcluster)  [unwired: 8 in, 1 out]
        n132 = local read "Scanning"() -> (w226:T26)
        n133 = local read "B-Scans Per Buffer"() -> (w227:i32)
        n134 = call "galvo_functional_global.vi"("Est Sweep Speed"=w227, "State"=galvo_states."Load Raster", "error in (no error)"=w224, "user event out"=w226) -> ("error out"=w223:errorcluster)  [unwired: 6 in, 1 out]
        n135 = Enqueue Element(queue=w235, element=OCT_Hardware_States."Initialize DAQ", error in (no error)=w223) -> (queue out=w232:refnum<queue>, error out=w231:errorcluster)  [unwired: 1 in, 1 out]
        n136 = local read "Save Data"() -> (w230:bool)
        n137 = case shown="False" w230 {
          tunnel: w232 -> [w239 w244]
          tunnel: w231 -> [w238 w243]
          tunnel: [FALSE ("Reset DAQ") FALSE ("Reset DAQ")] -> w229
          frame False {
            n138 = Enqueue Element(queue=w239, element=OCT_Hardware_States."Acquire Data", error in (no error)=w238) -> ()  [unwired: 1 in, 3 out]
          }
          frame True {
            n139 = Enqueue Element(queue=w244, element=OCT_Hardware_States."Acquire Data", error in (no error)=w243) -> ()  [unwired: 1 in, 3 out]
          }
        }
        n140 = local write "Save Data"(w229) -> ()
      }
      frame "Stop" {
        n141 = flat-sequence {
          tunnel: w251 -> [w262]
          tunnel: [w262] -> w250
          frame #0 {
            n142 = local write "Processing Finished"(FALSE ("Reset DAQ")) -> ()
            n143 = local write "Reset DAQ"(FALSE ("Reset DAQ")) -> ()
          }
        }
        n144 = call "Save Data Functional Global.vi"("States"=Saving_Data_States."Flush Queue", "error in (no error)"=w250) -> ("error out"=w255:errorcluster)  [unwired: 6 in, 3 out]
        n145 = call "OCT Processing 2ch functional global.vi"("State"=processing_states."Flush Data", "error in (no error)"=w255) -> ("error out"=w247:errorcluster)  [unwired: 5 in, 4 out]
        n146 = property on="Save Sweep" class="Bool"(error in=w247, "DisabledEnum"=T35."Disabled and Grayed Out" ("Disabled")) -> (error out=w246:errorcluster)  [unwired: 1 in, 1 out]
        n147 = Enqueue Element(queue=w253, element=OCT_Hardware_States."Save Sweep", error in (no error)=w246) -> (error out=w249:errorcluster)  [unwired: 1 in, 2 out]
        n148 = flat-sequence {
          tunnel: w249 -> [_]
          frame #0 {
            w260 = 0 ("DeviceIn")
            n149 = call "ATS_AsyncDMA_Device.vi"("DeviceIn"=w260, "ATS_Async_Ctrl"=ATS_Async_Ctrl."Stop") -> ("ReadSamples_Out"=w259:T37)  [unwired: 9 in, 4 out]
            n150 = call "ATS_AsyncDMA_Device.vi"("DeviceIn"=w260, "ATS_Async_Ctrl"=ATS_Async_Ctrl."Abort", "ReadSamples"=w259) -> ()  [unwired: 8 in, 5 out]
          }
        }
      }
      frame "Save Sweep" {
        # "Gage if you need\nthe gage card,\nenable here"
        n151 = case shown="True" TRUE {
          tunnel: w264 -> [_ w266]
          frame False {
          }
          frame True {
            w270 = 0 ("DeviceIn")
            n152 = local read "Clock Length"() -> (w272:u32)
            n153 = local read "Async_Setting"() -> (w268:T1)
            n154 = Bundle By Name(cluster=w268, "UseHeader"=u32 0, "Rec/Buffer"=u32 125, "Total_Rec"=u32 0) -> (w269:T1)
            n155 = Unbundle By Name(w266) -> ("Record.Presize"=w273:u32)
            n156 = Bundle By Name(cluster=T37 {"Offset"=0, "Length"=0} ("ReadSamples"), "Length"=w272, "Offset"=w273) -> (w271:T37)
            n157 = call "ATS_AsyncDMA_Device.vi"("DeviceIn"=w270, "ATS_Async_Ctrl"=ATS_Async_Ctrl."SetupDMA" ("ATS_DMA_Ctrl"), "Async_Mode"=ATS_Async_Mode."Traditional", "Async_Setting"=w269, "Channel"=ATS_DMA_Channel."Channel_B", "ReadSamples"=w271, "Start Now / Wait"=TRUE) -> ("Buffer"=w278:u16[])  [unwired: 4 in, 4 out]
            n158 = while {
              tunnel: w278 -> [_]
              shift-right: [ATS_Async_Ctrl."Get" ("ATS_Async_Ctrl")] -> _
              shift-left: ATS_Async_Ctrl."StartCapture" ("ATS_Async_Ctrl") -> [w292]
              tunnel: w270 -> [w286]
              stop <- w289 stop-if-true
              n159 = call "ATS_AsyncDMA_Device.vi"("DeviceIn"=w286, "ATS_Async_Ctrl"=w292) -> ("Buffer"=w284:u16[], "Async_Status"=w283:T5)  [unwired: 9 in, 3 out]
              n160 = Unbundle By Name(w283) -> ("Valid"=w285:bool, "Completed"=w294:bool, "Start DMA"=w295:bool, "Timeout"=w296:bool, "Error"=w293:bool)
              n161 = property on="Reset DAQ" class="Bool (strict)"() -> ("Value"=w290:bool)  [unwired: 2 in, 2 out]
              n162 = local read "Clock Length"() -> (w287:u32)
              n163 = Compound Arithmetic op=OR(w294, invert w295, w296, w293, w290) -> (w288:bool)
              n164 = case shown="True" w285 {
                selector: w285 -> [w297 w300]
                tunnel: w284 -> [_ w299]
                tunnel: [w297 w300] -> w289
                tunnel: w288 -> [_ _]
                tunnel: w287 -> [_ w298]
                frame False {
                }
                frame True {
                  n165 = Array Subset(array=w299, length=w298) -> (w301:u16[])  [unwired: 1 in]
                  n166 = call "Clock Frequency generator hilbert.vi"(7:6300.0 ("Sweep Speed"), "Acquisition speed (S/s)"=180000000.0 ("Sweep Speed"), "k-space signal in"=w301, "number of frequency updates"=4385) -> ("Error Out"=w306:errorcluster, "frequency\nsteps"=w305:i32)  [unwired: 6 in]
                  n167 = call "wavepond sequence.vi"("Error In"=w306, "Number of updates"=w305) -> ()  [unwired: 9 in, 1 out]
                }
              }
            }
          }
        }
      }
      frame "Initialize DAQ" {
        # "B-Scans per buffer should be around 4 if \ntaking more than 1 to minimize data transfer"
        # "If B Scans is 1, set total records to 0,\notherwise it should be A-Scans Per\nBScan times BScans"
        # "BScans Per Buffer"
        n168 = local read "First Time?"() -> (w311:bool)
        n169 = case shown="False" w311 {
          tunnel: [_ w343] -> w337
          tunnel: w314 -> [_ w339]
          tunnel: [FALSE ("First Time?") FALSE ("First Time?")] -> w310
          frame False {
          }
          frame True {
            n170 = call "ATS_Device.vi"("BoardToVerify"=w339, "ATS_Check"=ATS_Check_Ctrl."Verify Board", "DevCtrl"=Device_Ctrl."Initialize", "DeviceIn"=0 ("Device")) -> ("error out"=w341:errorcluster, "DeviceOut"=w345:i32)  [unwired: 1 in, 5 out]
            n171 = call "ATS_Device.vi"("error in (no error)"=w341, "DevCtrl"=Device_Ctrl."Abort", "DeviceIn"=w345) -> ("DeviceOut"=w343:i32)  [unwired: 2 in, 6 out]
          }
        }
        n172 = local write "First Time?"(w310) -> ()
        n173 = Unbundle By Name(w307) -> ("Record.Length"=w315:u32)
        n174 = call "ATS_MS_Set_Device.vi"("Set_Manually (F)"=FALSE, "Setup_In"=w307, "DeviceIn"=w337) -> ("Setup_Out"=w308:T7)  [unwired: 3 in, 5 out]
        n175 = local read "Scanning"() -> (w333:T26)
        n176 = Unbundle By Name(w333) -> ("B-scans (rings)"=w321:u32, "A(cluster)/B"=w331:u32, "B-scans (rings)"=w326:u32, "A(cluster)/B"=w325:u32, "B-scans (rings)"=w323:u32, "A(cluster)/B"=w317:u32)
        n177 = Not Equal?(x=w323, y=u32 1 ("x")) -> (x != y?=w324:bool)
        n178 = Equal?(x=u32 1, y=w321) -> (x = y?=w327:bool)
        n179 = local read "B-Scans Per Buffer"() -> (w309:i32)
        n180 = Select(t=u32 4 ("y"), s=w327, f=w309) -> (s? t:f=w329:u32)
        n181 = Multiply(x=w326, y=w325) -> (x*y=w320:u32)
        n182 = local read "Async_Setting"() -> (w313:T1)
        n183 = Select(t=w320, s=w324, f=u32 0 ("Total_Rec")) -> (s? t:f=w335:u32)
        n184 = Multiply(x=w329, y=w331) -> (x*y=w332:u32)
        n185 = Bundle By Name(cluster=T6 {"Points Per A-Scan"=0, "A-Scans per B-Scan"=0, "Voltage Range"=4.0, "Card Resolution (bits)"=16} ("Imaging Parameters"), "Points Per A-Scan"=w315, "A-Scans per B-Scan"=w317) -> (w316:T6)
        n186 = Bundle By Name(cluster=w313, "UseHeader"=u32 0, "Rec/Buffer"=w332, "Total_Rec"=w335) -> (w312:T1)
        n187 = local write "Async_Setting"(w312) -> ()
        n188 = local write "Imaging Parameters"(w316) -> ()
      }
      frame "Acquire Data", Default {
        w370 = 0 ("DeviceIn")
        # "Update and \nclear the \nEn Face"
        # "Tell the FFT the most\nup-to-date imaging\nparameters"
        n189 = Enqueue Element(queue=w362, element=OCT_Hardware_States."Stop", error in (no error)=w353) -> (error out=w352:errorcluster)  [unwired: 1 in, 2 out]
        n190 = local read "Imaging Parameters"() -> (w359:T6)
        n191 = local read "Data Format"() -> (w364:T23)
        n192 = local read "Async_Setting"() -> (w357:T1)
        n193 = case shown="\"Channel 1\", Default" w364 {
          tunnel: [ATS_DMA_Channel."Channel_A" ("Channel") ATS_DMA_Channel."A & B" ("Channel") ATS_DMA_Channel."A & B" ("Channel")] -> w363
          frame "Channel 1", Default {
          }
          frame "Channel 2" {
          }
          frame "Channel 1 and 2" {
          }
        }
        n194 = call "OCT Processing 2ch functional global.vi"("State"=processing_states."Update Imaging Parameters", "error in (no error)"=w352, "Input Parameters"=w359) -> ("error out"=w361:errorcluster)  [unwired: 4 in, 4 out]
        n195 = local read "Scanning"() -> (w356:T26)
        n196 = call "En Face Functional Global.vi"(7:En_Face_States."Clear En Face" ("En Face States"), "Error In"=w361, 9:w356) -> ("Error Out"=w355:errorcluster)  [unwired: 7 in, 1 out]
        n197 = Unbundle By Name(w349) -> ("Record.Length"=w366:u32, "Record.Presize"=w365:u32)
        n198 = Unbundle By Name(w349) -> ("Record.Length"=w348:u32)
        n199 = call "OCT Processing 2ch functional global.vi"("State"=processing_states."Get Queue", "error in (no error)"=w355) -> ("queue out"=w351:refnum<queue>)  [unwired: 5 in, 4 out]
        n200 = Bundle By Name(cluster=T37 {"Offset"=0, "Length"=0} ("ReadSamples"), "Length"=w366, "Offset"=w365) -> (w372:T37)
        n201 = call "ATS_AsyncDMA_Device.vi"("DeviceIn"=w370, "ATS_Async_Ctrl"=ATS_Async_Ctrl."SetupDMA" ("ATS_DMA_Ctrl"), "Async_Mode"=ATS_Async_Mode."No-Pre-Trigger", "Async_Setting"=w357, "Channel"=w363, "ReadSamples"=w372, "Start Now / Wait"=TRUE) -> ("Buffer"=w368:u16[])  [unwired: 4 in, 4 out]
        n202 = while {
          tunnel: w368 -> [_]
          tunnel: w370 -> [w396]
          shift-right: [ATS_Async_Ctrl."Get" ("ATS_Async_Ctrl")] -> _
          shift-left: ATS_Async_Ctrl."StartCapture" ("ATS_Async_Ctrl") -> [w393]
          tunnel: w351 -> [w385]
          tunnel: [w384] -> w350
          tunnel: w348 -> [w383]
          stop <- w384 stop-if-true
          n203 = call "ATS_AsyncDMA_Device.vi"("DeviceIn"=w396, "ATS_Async_Ctrl"=w393) -> ("Buffer"=w389:u16[], "Async_Status"=w391:T5)  [unwired: 9 in, 3 out]
          "Async_Status" <- w391
          n204 = Unbundle By Name(w391) -> ("Valid"=w390:bool, "Completed"=w386:bool, "Start DMA"=w387:bool, "Timeout"=w395:bool, "Error"=w394:bool)
          n205 = local read "Reset DAQ"() -> (w388:bool)
          n206 = Compound Arithmetic op=OR(w386, invert w387, w395, w394, w388) -> (w384:bool)
          n207 = case shown="True" w390 {
            tunnel: w389 -> [_ w401]
            tunnel: w385 -> [_ w403]
            tunnel: w383 -> [_ w400]
            frame False {
              # "Do nothing"
            }
            frame True {
              n208 = Enqueue Element(queue=w403, element=w401, timeout in ms (-1)=50) -> (error out=w398:errorcluster)  [unwired: 1 in, 2 out]
              n209 = property on="Save Sweep" class="Bool"(error in=w398, "DisabledEnum"=T35."Enabled" ("Disabled")) -> ()  [unwired: 1 in, 2 out]
              n210 = call "Display Raw Data.vi"("Enum"=Display_Raw_Data_states."Add Processed", "Length"=w400, "Raw Data In"=w401) -> ()  [unwired: 9 in]
            }
          }
        }
        n211 = while {
          tunnel: w350 -> [w379]
          stop <- w377 stop-if-true
          n212 = local read "Processing Finished"() -> (w378:bool)
          n213 = Wait (ms)(milliseconds to wait=u32 50) -> ()  [unwired: 1 out]
          n214 = And(x=w379, y=w378) -> (x .and. y?=w377:bool)
        }
      }
      frame "Acquire Data" {
        w431 = 0 ("DeviceIn")
        # "Close files and set save \nstate to do nothing"
        # "Update and \nclear the \nEn Face"
        # "Tell the FFT the most\nup-to-date imaging\nparameters"
        n215 = local read "Imaging Parameters"() -> (w420:T6)
        n216 = local read "Data Format"() -> (w425:T23)
        n217 = local read "Async_Setting"() -> (w414:T1)
        n218 = case shown="\"Channel 1\", Default" w425 {
          tunnel: [ATS_DMA_Channel."Channel_A" ("Channel") ATS_DMA_Channel."A & B" ("Channel") ATS_DMA_Channel."A & B" ("Channel")] -> w424
          frame "Channel 1", Default {
          }
          frame "Channel 2" {
          }
          frame "Channel 1 and 2" {
          }
        }
        n219 = call "OCT Processing 2ch functional global.vi"("State"=processing_states."Update Imaging Parameters", "error in (no error)"=w406, "Input Parameters"=w420) -> ("error out"=w422:errorcluster)  [unwired: 4 in, 4 out]
        n220 = local read "Scanning"() -> (w413:T26)
        n221 = call "En Face Functional Global.vi"(7:En_Face_States."Clear En Face" ("En Face States"), "Error In"=w422, 9:w413) -> ("Error Out"=w412:errorcluster)  [unwired: 7 in, 1 out]
        n222 = Unbundle By Name(w404) -> ("Record.Length"=w427:u32, "Record.Presize"=w426:u32)
        n223 = call "Save Data Functional Global.vi"("States"=Saving_Data_States."Get Queue", "error in (no error)"=w406) -> ("Saving Queue Out"=w407:refnum<queue>)  [unwired: 6 in, 3 out]
        n224 = call "OCT Processing 2ch functional global.vi"("State"=processing_states."Get Queue", "error in (no error)"=w412) -> ("error out"=w411:errorcluster, "queue out"=w409:refnum<queue>)  [unwired: 5 in, 3 out]
        n225 = Bundle By Name(cluster=T37 {"Offset"=0, "Length"=0} ("ReadSamples"), "Length"=w427, "Offset"=w426) -> (w433:T37)
        n226 = call "ATS_AsyncDMA_Device.vi"("DeviceIn"=w431, "ATS_Async_Ctrl"=ATS_Async_Ctrl."SetupDMA" ("ATS_DMA_Ctrl"), "Async_Mode"=ATS_Async_Mode."No-Pre-Trigger", "Async_Setting"=w414, "Channel"=w424, "ReadSamples"=w433, "Start Now / Wait"=TRUE) -> ("Buffer"=w429:u16[])  [unwired: 4 in, 4 out]
        n227 = while {
          tunnel: w411 -> [_]
          tunnel: [w442] -> w419
          i -> [w441]
          stop <- w440 stop-if-true
          # "Saves data as long as data is being fed into the Queue,\notherwise it will time out and halt this loop."
          n228 = case shown="1, Default" w441 {
            tunnel: [FALSE w448] -> w440
            tunnel: [_ w445] -> w442
            frame 0 {
              # "Wait for data to Q up"
              n229 = Wait (ms)(milliseconds to wait=u32 1000) -> ()  [unwired: 1 out]
            }
            frame 1, Default {
              n230 = local read "Data Format"() -> (w451:T23)
              n231 = call "Save Data Functional Global.vi"("States"=Saving_Data_States."Save Data", "Data Format"=w451) -> ("error out"=w446:errorcluster)  [unwired: 6 in, 3 out]
              n232 = call "Save Data Functional Global.vi"("States"=Saving_Data_States."Get Queue Size", "error in (no error)"=w446) -> ("error out"=w445:errorcluster, "# elements in queue"=w447:i32)  [unwired: 6 in, 2 out]
              n233 = Equal To 0?(x=w447) -> (x = 0?=w448:bool)
            }
          }
        }
        n234 = while {
          tunnel: w429 -> [_]
          tunnel: w431 -> [w465]
          shift-right: [ATS_Async_Ctrl."Get" ("ATS_Async_Ctrl")] -> _
          shift-left: ATS_Async_Ctrl."StartCapture" ("ATS_Async_Ctrl") -> [w462]
          tunnel: w409 -> [w454]
          tunnel: w407 -> [w453]
          stop <- w452 stop-if-true
          n235 = call "ATS_AsyncDMA_Device.vi"("DeviceIn"=w465, "ATS_Async_Ctrl"=w462) -> ("Buffer"=w458:u16[], "Async_Status"=w460:T5)  [unwired: 9 in, 3 out]
          n236 = Unbundle By Name(w460) -> ("Valid"=w459:bool, "Completed"=w455:bool, "Start DMA"=w456:bool, "Timeout"=w464:bool, "Error"=w463:bool)
          n237 = local read "Reset DAQ"() -> (w457:bool)
          n238 = Compound Arithmetic op=OR(w455, invert w456, w464, w463, w457) -> (w452:bool)
          n239 = case shown="True" w459 {
            tunnel: w458 -> [_ w468]
            tunnel: w458 -> [_ w469]
            tunnel: w454 -> [_ w470]
            tunnel: w453 -> [_ w467]
            frame False {
              # "Do nothing"
            }
            frame True {
              w466 = 50 ("timeout in ms (-1)")
              n240 = Enqueue Element(queue=w467, element=w468, timeout in ms (-1)=w466) -> ()  [unwired: 1 in, 3 out]
              n241 = Enqueue Element(queue=w470, element=w469, timeout in ms (-1)=w466) -> ()  [unwired: 1 in, 3 out]
            }
          }
        }
        n242 = call "Save Data Functional Global.vi"("States"=Saving_Data_States."Close Files", "error in (no error)"=w419) -> ("error out"=w418:errorcluster)  [unwired: 6 in, 3 out]
        n243 = call "Save Data Functional Global.vi"("States"=Saving_Data_States."Do Nothing" ("Save State"), "error in (no error)"=w418) -> ("error out"=w416:errorcluster)  [unwired: 6 in, 3 out]
        n244 = Enqueue Element(queue=w423, element=OCT_Hardware_States."Stop", error in (no error)=w416) -> ()  [unwired: 1 in, 3 out]
      }
      frame "Set Resampling Array" {
        n245 = Wait (ms)(milliseconds to wait=u32 10) -> ()  [unwired: 1 out]
      }
      frame "Stop" {
        n246 = Release Queue(queue=w482, error in (no error)=w481) -> (error out=w480:errorcluster)  [unwired: 1 in, 2 out]
        n247 = call "OCT Processing 2ch functional global.vi"("State"=processing_states."Shutdown", "error in (no error)"=w480) -> ("error out"=w479:errorcluster)  [unwired: 5 in, 4 out]
        n248 = call "Save Data Functional Global.vi"("States"=Saving_Data_States."Shutdown", "error in (no error)"=w479) -> ("error out"=w476:errorcluster)  [unwired: 6 in, 3 out]
        n249 = call "galvo_functional_global.vi"("State"=galvo_states."Shutdown", "error in (no error)"=w476) -> ("error out"=w475:errorcluster)  [unwired: 8 in, 1 out]
        n250 = flat-sequence {
          tunnel: w475 -> [_]
          frame #0 {
            w486 = 0 ("DeviceIn")
            n251 = call "ATS_AsyncDMA_Device.vi"("DeviceIn"=w486, "ATS_Async_Ctrl"=ATS_Async_Ctrl."Stop") -> ("ReadSamples_Out"=w485:T37)  [unwired: 9 in, 4 out]
            n252 = call "ATS_AsyncDMA_Device.vi"("DeviceIn"=w486, "ATS_Async_Ctrl"=ATS_Async_Ctrl."Abort", "ReadSamples"=w485) -> ()  [unwired: 8 in, 5 out]
          }
          frame #1 {
            n253 = Stop(stop? (T)=TRUE) -> ()
          }
        }
      }
      frame "Set Clock" {
        w491 = T15 12 items=["20mV", "40mV", "50mV", "80mV", "100mV", "200mV", "400mV", "500mV", "800mV", "1 V", "1.25 V", "2 V", "4 V", "5 V", "8 V", "10 V", "16 V", "20 V", "40 V", "HiFi"] ("Input B.Range")
        w494 = u32 18 items=["1 kS/s", "2 kS/s", "5 kS/s", "10 kS/s", "20 kS/s", "50 kS/s", "100 kS/s", "200 kS/s", "500 kS/s", "1 MS/s", "2 MS/s", "5 MS/s", "10 MS/s", "20 MS/s", "50 MS/s", "100 MS/s", "125 MS/s", "160 MS/s", "180 MS/s"] ("ClckRate")
        n254 = local read "Clock Length"() -> (w493:u32)
        n255 = call "ATS_Device.vi"("BoardToVerify"=w489, "ATS_Check"=ATS_Check_Ctrl."Verify Board", "DevCtrl"=Device_Ctrl."Initialize", "DeviceIn"=0 ("Device")) -> ("error out"=w496:errorcluster, "DeviceOut"=w501:i32)  [unwired: 1 in, 5 out]
        n256 = Bundle By Name(cluster=w488, "Record.Length"=w493, "Clock.ClckSource"=ClockSource."Internal", "Clock.ClckRate"=w494, "Input B.Range"=w491, "Input A.Impedance"=Impedance."50 ohms") -> (w492:T7)
        n257 = call "ATS_Device.vi"("error in (no error)"=w496, "DevCtrl"=Device_Ctrl."Abort", "DeviceIn"=w501) -> ("DeviceOut"=w499:i32)  [unwired: 2 in, 6 out]
        n258 = call "ATS_MS_Set_Device.vi"("Set_Manually (F)"=FALSE, "Setup_In"=w492, "DeviceIn"=w499) -> ()  [unwired: 3 in, 6 out]
      }
    }
  }
  n259 = Destroy User Event(user event=w10) -> ()  [unwired: 1 in, 1 out]
